vi "SpreadsheetStorage.vi"() -> ()   [LabVIEW 2014]
uses:
  <vilib>/Utility/file.llb/Write To Spreadsheet File (DBL).vi
panel:
  in  "Wave Parameters":T1 {"Amplitude" format="%#_13g"; "Signal Frequency" format="%#_13g"}
  in  "Digitizing Parameters":T2 {"Sampling Frequency" format="%#_13g"; "Number of Samples" format="%#_13g"}
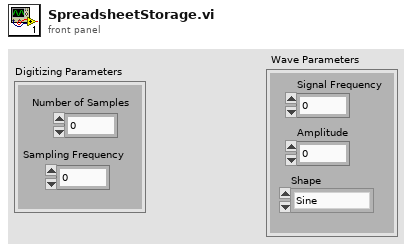
[diagram p1: front panel]
types:
  T1 = cluster{"Signal Frequency":dbl, "Amplitude":dbl, "Shape":enum16{"Sine", "Cosine", "DC Level", "Square", "User Defined"}}
  T2 = cluster{"Number of Samples":dbl, "Sampling Frequency":dbl}
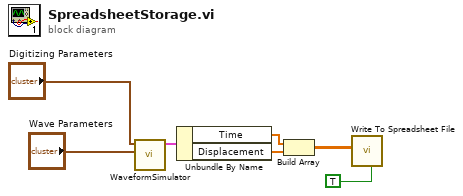
[diagram p0: block diagram]
diagram:
  n1 = call "WaveformSimulator.vi"("Wave Parameters"="Wave Parameters", "Digitizing Parameters"="Digitizing Parameters") -> ("Waveform Output"=w3:cluster{"Time":dbl[], "Displacement":dbl[]})  [unwired: 7 in]
  n2 = Unbundle By Name(w3) -> ("Time"=w2:dbl[], "Displacement"=w1:dbl[])
  n3 = Build Array(w2, w1) -> (w6:dbl[][])
  n4 = call-poly <vilib>:"Write To Spreadsheet File.vi"("transpose? (no:F)"=TRUE, "2D data"=w6) -> ()  [unwired: 6 in, 1 out]
